vi "randn_approximation.vi"(2 "N":i32=1) -> (0 "randn() vector":dbl[](array[numeric]))   [LabVIEW 2020]
doc: "Normal distribution random number generator using Marsaglia polar method. Std is 1, mean is 0."
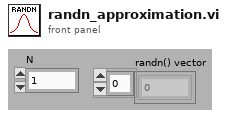
[diagram p1: front panel]
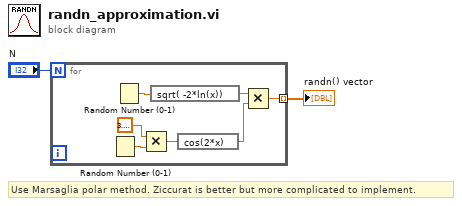
[diagram p0: block diagram]
diagram:
  # "Use Marsaglia polar method. Ziccurat is better but more complicated to implement."
  n1 = for {
    N: "N" -> [_]
    tunnel: [w3] -> w1 mode=indexing
    n2 = Random Number (0-1)() -> (number: 0 to 1=w7:dbl)
    n3 = Random Number (0-1)() -> (number: 0 to 1=w9:dbl)
    n4 = Multiply(x=3.141592653589793, y=w7) -> (x*y=w8:dbl)
    n5 = expression code="sqrt( -2*ln(x))"(w9) -> (w4:dbl)
    n6 = expression code="cos(2*x)"(w8) -> (w5:dbl)
    n7 = Multiply(x=w4, y=w5) -> (x*y=w3:dbl)
  }
  "randn() vector" <- w1
